vi "GetWheelLocations (SubVI).vi"(10 "robotWheelbaseXLength(m)":dbl, 11 "robotWheelbaseYLength(m)":dbl) -> (3 "wheelLocations":T1[](array[typedef]) {"Y" format="%14.3f"; "X" format="%14.3f"})   [LabVIEW 2020]
uses:
  <vilib>/Rock Robotics/WPI/ThirdParty/JAS_Junk/TrajLib/TRANSLATION2D.ctl
  <vilib>/Rock Robotics/WPI/ThirdParty/JAS_Junk/TrajLib/Trajectory_Library.lvlib
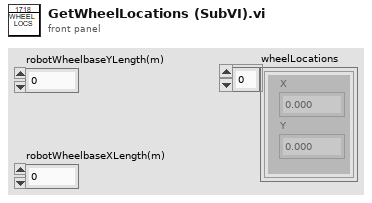
[diagram p1: front panel]
types:
  T1 = typedef "Trajectory_Library.lvlib/TRANSLATION2D.ctl" = cluster{"X":dbl, "Y":dbl}
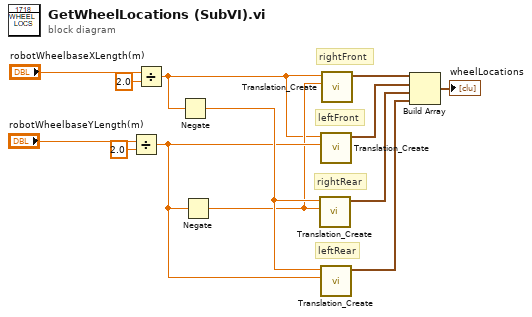
[diagram p0: block diagram]
diagram:
  # "rightRear"
  # "leftRear"
  # "rightFront"
  # "leftFront"
  n1 = Divide(x="robotWheelbaseYLength(m)", y=2.0) -> (x/y=w8:dbl)
  n2 = Divide(x="robotWheelbaseXLength(m)", y=2.0) -> (x/y=w6:dbl)
  n3 = Negate(x=w6) -> (-x=w9:dbl)
  n4 = Negate(x=w8) -> (-x=w7:dbl)
  n5 = call <vilib>:"Translation_Create.vi"("Y"=w7, "X"=w9) -> ("TRANSLATION"=w12:T1)  [unwired: 9 in]
  n6 = call <vilib>:"Translation_Create.vi"("Y"=w8, "X"=w6) -> ("TRANSLATION"=w11:T1)  [unwired: 9 in]
  n7 = call <vilib>:"Translation_Create.vi"("Y"=w8, "X"=w9) -> ("TRANSLATION"=w13:T1)  [unwired: 9 in]
  n8 = call <vilib>:"Translation_Create.vi"("Y"=w7, "X"=w6) -> ("TRANSLATION"=w10:T1)  [unwired: 9 in]
  n9 = Build Array(w10, w11, w12, w13) -> (→"wheelLocations":T1[])
